vi "DevB.Close Session.vi"(8 "error in (no error)":errorcluster, 11 "DevB Session":T1) -> (0 "error out":errorcluster)   [LabVIEW 2018]
uses:
  typedefs/DevB.Session.ctl
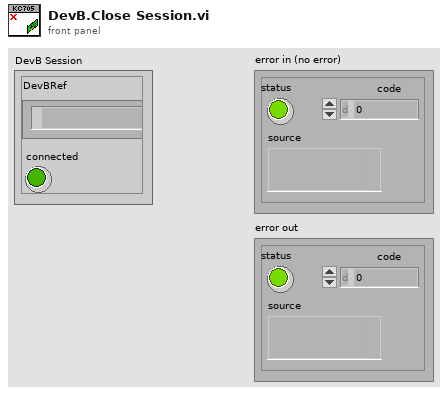
[diagram p1: front panel]
types:
  T1 = typedef "DevB.Session.ctl" = cluster{"DevBRef":refnum<visa-resource-name>, "connected":bool}
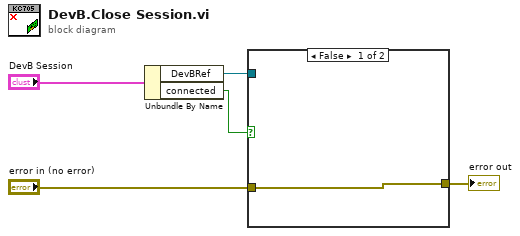
[diagram p0: block diagram]
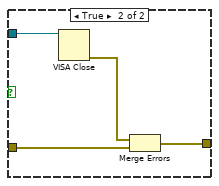
[diagram p2: hidden frame]
diagram:
  n1 = Unbundle By Name("DevB Session") -> ("DevBRef"=w4:refnum<visa-resource-name>, "connected"=w1:bool)
  n2 = case shown="False" w1 {
    tunnel: w4 -> [_ w10]
    tunnel: [w6 w9] -> w3
    tunnel: "error in (no error)" -> [w6 w8]
    frame False {
    }
    frame True {
      n3 = VISA Close(VISA resource name=w10) -> (error out=w7:errorcluster)  [unwired: 1 in]
      n4 = Merge Errors(w7, w8) -> (w9:errorcluster)
    }
  }
  "error out" <- w3
